vi "CRYPEAQ gp.vi"(9 "W":dbl=32768.0, 10 "NF":dbl=92.0, 11 "fcN":dbl=1019.5) -> (3 "gp":dbl)   [LabVIEW 2013]
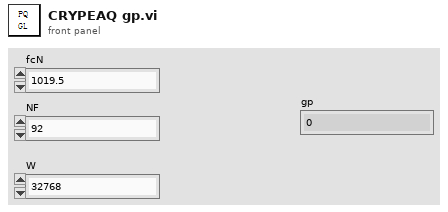
[diagram p1: front panel]
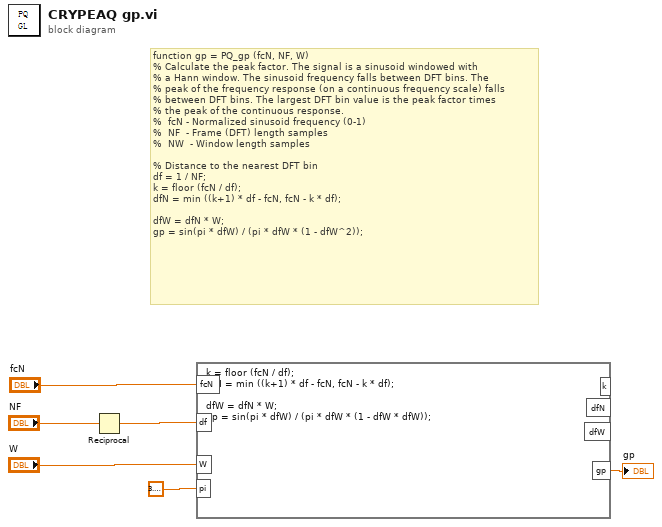
[diagram p0: block diagram]
diagram:
  # "function gp = PQ_gp (fcN, NF, W)\n% Calculate the peak factor. The signal is a sinusoid windowed with\n% a Hann window. The sinusoid frequency falls between DFT bins. The\n% peak of the frequency response (on a continuous frequency scale) falls\n% between DFT bins. The largest DFT bin value is the peak factor times\n% the peak of the continuous response.\n%  fcN - Normalized sinusoid frequency (0-1)\n%  NF  - Frame (DFT) length samples\n%  NW  - Window length samples\n\n% Distance to the nearest DFT bin\ndf = 1 / NF;\nk = floor (fcN / df);\ndfN = min ((k+1) * df - fcN, fcN - k * df);\n\ndfW = dfN * W;\ngp = sin(pi * dfW) / (pi * dfW * (1 - dfW^2));"
  n1 = Reciprocal(x="NF") -> (1/x=w3:dbl)
  n2 = formula code="k = floor (fcN / df);\ndfN = min ((k+1) * df - fcN, fcN - k * df);\n\ndfW = dfN * W;\ngp = sin(pi * dfW) / (pi * dfW * (1 - dfW * dfW));"("W"="W", "df"=w3, "fcN"="fcN", "pi"=3.141592653589793) -> ("gp"=→"gp":dbl)  [unwired: 3 out]
